vi "generateInternalShutdown.vi"(8 "error in (no error)":errorcluster, 10 "ShutdownEvent":T1, 11 "UserEvents in":refnum<class "UserEvents.lvclass">) -> (0 "error out":errorcluster, 3 "UserEvents out":refnum<class "UserEvents.lvclass">)   [LabVIEW 2016, in "UserEvents.lvclass"]
uses:
  UserEvents.lvclass
  DataTypes/General/ShutdownEvent.ctl
  UserEvents.lvclass/UserEvents.ctl
  DataTypes/General/M1M3SupportGeneral.lvlib
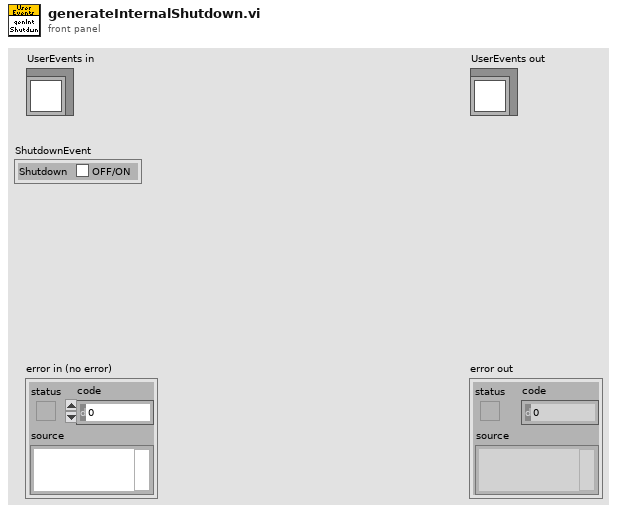
[diagram p1: front panel]
types:
  T1 = typedef "M1M3SupportGeneral.lvlib/ShutdownEvent.ctl" = cluster{"Shutdown":bool}
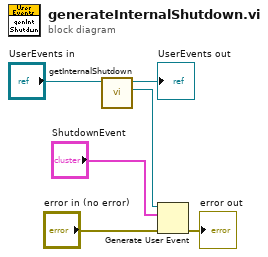
[diagram p0: block diagram]
diagram:
  n1 = call "getInternalShutdown.vi"("UserEvents in"="UserEvents in") -> ("InternalShutdown"=w5:refnum<user-event>, "UserEvents out"=→"UserEvents out":refnum<class "UserEvents.lvclass">)  [unwired: 9 in]
  n2 = Generate User Event(user event=w5, event data cluster="ShutdownEvent", error in="error in (no error)") -> (error out=→"error out":errorcluster)  [unwired: 1 in, 1 out]
